vi "FPGA_Main_v8.vi"() -> ()   [LabVIEW 2018]
uses:
  <instrlib>/_niInstr/Basic Elements/v1/FPGA/niInstr Basic Elements v1 FPGA.lvlib
  <instrlib>/_niInstr/Basic Elements/v1/FPGA/Private/Count Down U16.vi
  ctl/_FPGA_priRFSettings_Parameters.ctl
  <instrlib>/_niInstr/Basic Elements/v1/FPGA/Private/Count Down U32.vi
  <vilib>/rvi/DataTransferAndStorage/Container/XNode/niFpgaContainer.xnode
  <vilib>/rvi/DataTransferAndStorage/Register/Emulation/niFpgaRegisterEmulation.vi
panel:
  in  "RF Rst":bool
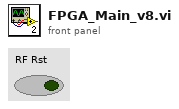
[diagram p1: front panel]
types:
  T1 = typedef "_FPGA_priRFSettings_Parameters.ctl" = cluster{"CycleIncrement":u32, "Amp":u32, "Total Ticks":u32, "Conj Ticks":u16, "Repeat":u16}
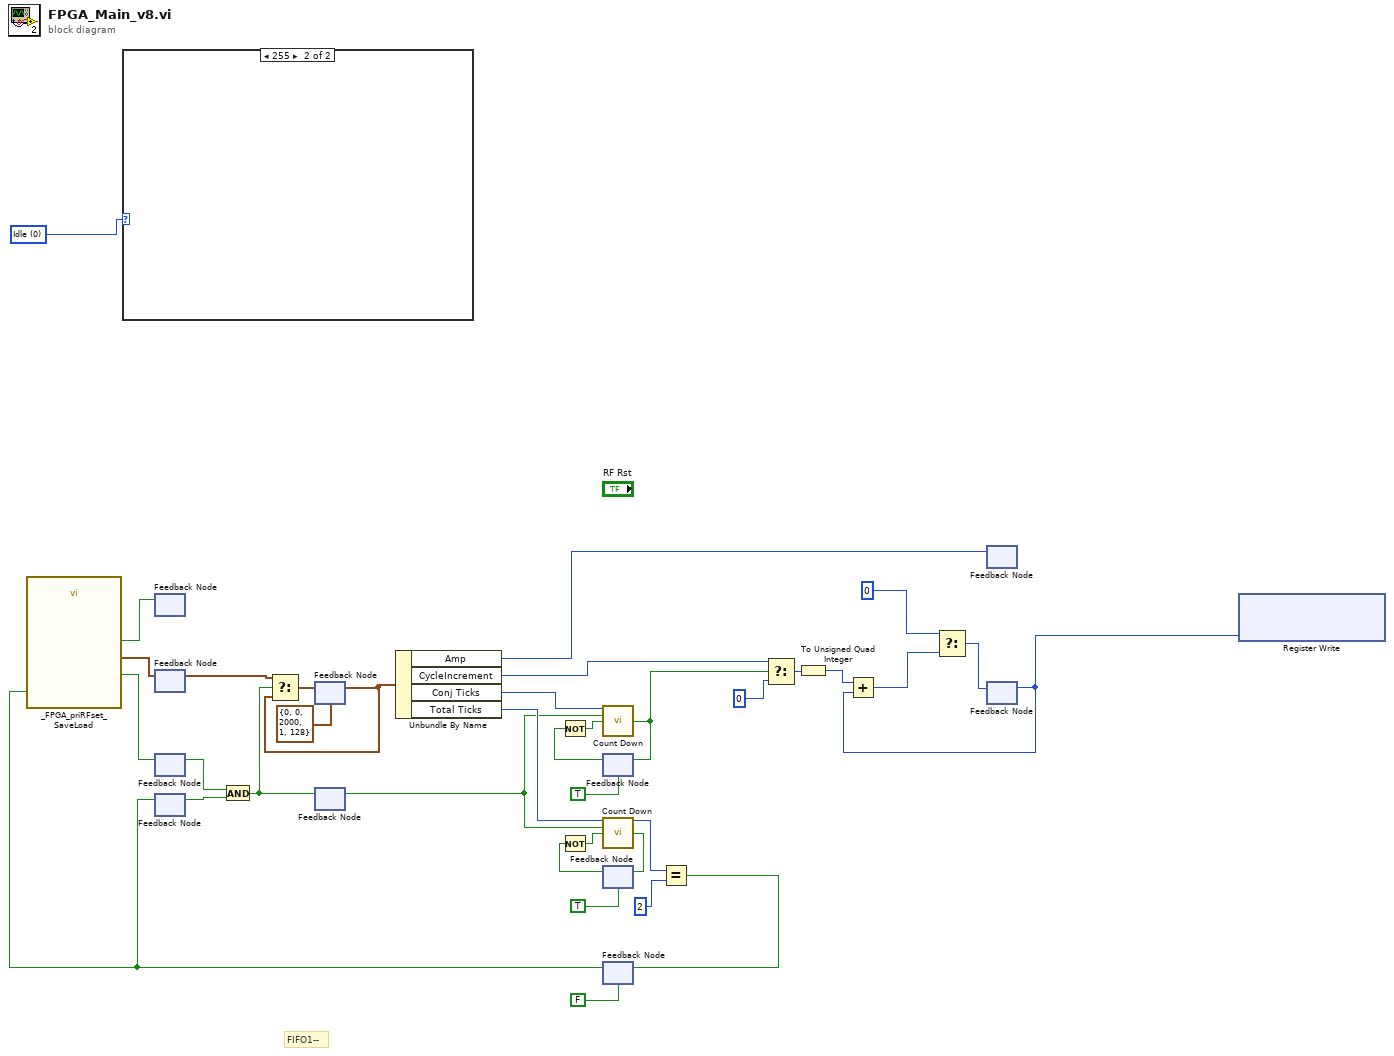
[diagram p0: block diagram]
diagram:
  w36 = u8 0 items=["Idle"=0, "EndofProcesses"=255]
  # "FIFO1--"
  n1 = case shown="255" w36 {
    frame 0, Default {
    }
    frame 255 {
    }
  }
  n2 = feedback #1() -> ()  [unwired: 2 in]
  n3 = feedback #2() -> (w4:T1)  [unwired: 1 in]
  n4 = feedback #3() -> (w3:bool)  [unwired: 1 in]
  n5 = feedback #4() -> (w2:bool)  [unwired: 1 in]
  n6 = And(x=w3, y=w2) -> (x .and. y?=w13:bool)
  n7 = feedback #5(T1 {"CycleIncrement"=0, "Amp"=0, "Total Ticks"=2000, "Conj Ticks"=1, "Repeat"=128} ("RF Set")) -> (w14:T1)
  n8 = Select(t=w4, s=w13, f=w14) -> (s? t:f=w34:T1)
  n9 = feedback-in #5(w34) -> ()
  n10 = feedback #6() -> (w11:bool)  [unwired: 1 in]
  n11 = feedback-in #6(w13) -> ()
  n12 = Unbundle By Name(w14) -> ("Amp"=w5:u32, "CycleIncrement"=w24:u32, "Conj Ticks"=w33:u16, "Total Ticks"=w20:u32)
  n13 = feedback #7(TRUE ("terminal count")) -> (w31:bool)
  n14 = Not(x=w31) -> (.not. x?=w30:bool)
  n15 = call-poly <instrlib>:"Count Down.vi"("count in"=w33, "load"=w11, "decrement"=w30) -> ("terminal count"=w25:bool)  [unwired: 11 in, 1 out]
  n16 = feedback-in #7(w25) -> ()
  n17 = feedback #8(TRUE ("terminal count")) -> (w27:bool)
  n18 = Not(x=w27) -> (.not. x?=w26:bool)
  n19 = call-poly <instrlib>:"Count Down.vi"("count in"=w20, "load"=w11, "decrement"=w26) -> ("count out"=w19:u32, "terminal count"=w28:bool)  [unwired: 11 in]
  n20 = feedback-in #8(w28) -> ()
  n21 = feedback #9(FALSE) -> (w15:bool)
  n22 = call "_FPGA_priRFset_SaveLoad.vi"("Load nxt"=w15) -> ("RF Set"=w35:T1, "First set?"=w7:bool, "CanLoad?"=w16:bool)  [unwired: 8 in]
  n23 = feedback-in #1(w7) -> ()
  n24 = feedback-in #2(w35) -> ()
  n25 = feedback-in #3(w16) -> ()
  n26 = feedback-in #4(w15) -> ()
  n27 = Equal?(x=w19, y=u32 2) -> (x = y?=w17:bool)
  n28 = feedback-in #9(w17) -> ()
  n29 = Select(t=w24, s=w25, f=u32 0) -> (s? t:f=w22:u32)
  n30 = To Unsigned Quad Integer(1:w22) -> (0:w21:u64)
  n31 = feedback #10() -> ()  [unwired: 2 in]
  n32 = feedback-in #10(w5) -> ()
  n33 = feedback #11() -> (w1:u64)  [unwired: 1 in]
  n34 = Add(x=w21, y=w1) -> (x+y=w10:u64)
  n35 = Select(t=u64 0, f=w10) -> (s? t:f=w9:u64)  [unwired: 1 in]
  n36 = feedback-in #11(w9) -> ()
  n37 = xnode "Register Write"("Data"=w1) -> ()  [unwired: 1 in, 1 out]
